vi "Launch Menu as Nested Panel.vi"(8 "error in (no error)":errorcluster, 11 "MainWindow in":refnum<class "MainWindow.lvclass">) -> (0 "error out":errorcluster, 3 "MainWindow out":refnum<class "MainWindow.lvclass">)   [LabVIEW 2020, in "MainWindow.lvlib" / "MainWindow.lvclass"]
uses:
  MainWindow.lvclass
  C:/Program Files (x86)/National Instruments/LabVIEW 2020/vi.lib/MGI/Panel Manager/Panel Actor/Panel Actor/Panel Actor.lvclass
  Menu/Menu/Menu.lvclass
  MainWindow.lvclass/MainWindow.ctl
  <vilib>/MGI/Panel Manager/Panel/Panel/Subpanel/Subpanel.lvclass
  C:/Program Files (x86)/National Instruments/LabVIEW 2020/vi.lib/MGI/Panel Manager/Panel/Panel/Panel.lvclass
  <vilib>/MGI/Panel Manager/Panel Actor/Panel Actor/Panel Actor.lvclass
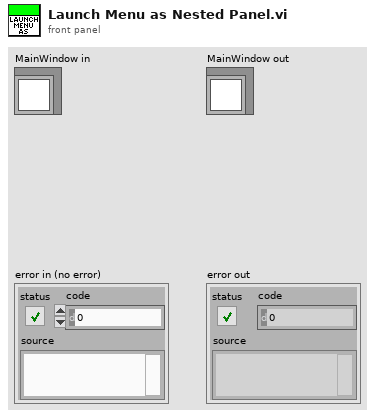
[diagram p1: front panel]
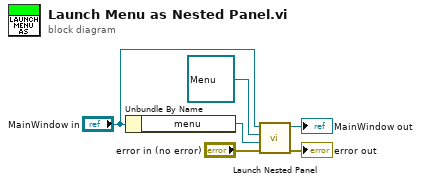
[diagram p0: block diagram]
diagram:
  n1 = Unbundle By Name("MainWindow in") -> ("menu"=w1:refnum<class "Subpanel.lvclass">)
  n2 = call <vilib>:"Launch Nested Panel.vi"("error in (no error)"="error in (no error)", "Panel"=w1, "Nested Panel Actor"=refnum<class "Menu.lvclass"> refnum ("Menu.lvlib:Menu.lvclass"), "Panel Actor in"="MainWindow in") -> ("error out"=→"error out":errorcluster, "Panel Actor in"=→"MainWindow out":refnum<class "MainWindow.lvclass">)  [unwired: 4 in, 2 out]
